vi "Init.vi"(8 "error in (no error)":errorcluster, 11 "Wifi in":refnum<class "Wifi.lvclass">) -> (0 "error out":errorcluster, 3 "Wifi out":refnum<class "Wifi.lvclass">)   [LabVIEW 2021, in "Wifi.lvclass"]
uses:
  Wifi.lvclass
  Wifi.lvclass/Wifi.ctl
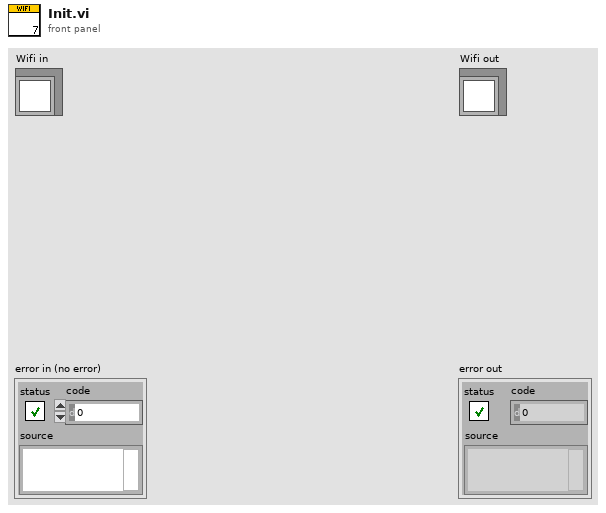
[diagram p1: front panel]
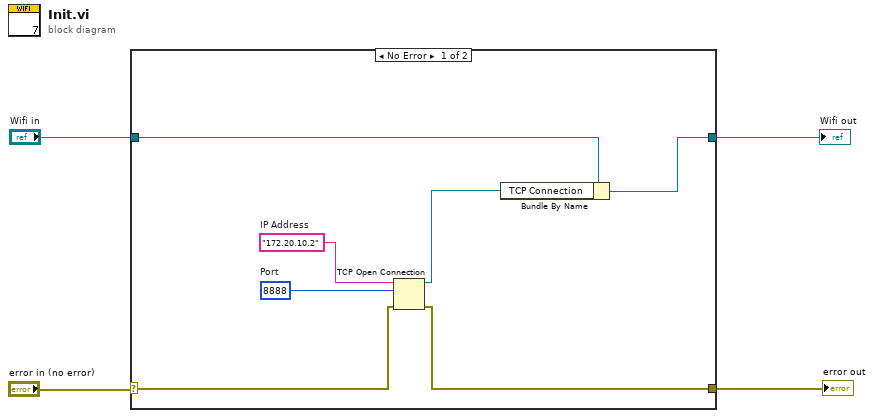
[diagram p0: block diagram]
diagram:
  n1 = case shown="No Error" "error in (no error)" {
    selector: "error in (no error)" -> [w9 w12]
    tunnel: [w8 w12] -> w3
    tunnel: [w5 w13] -> w2
    tunnel: "Wifi in" -> [w7 w13]
    frame No Error {
      w10 = u16 8888  # Port
      w11 = "172.20.10.2"  # IP Address
      n2 = TCP Open Connection(address=w11, remote port or service name=w10, error in (no error)=w9) -> (connection ID=w6:refnum<k5>, error out=w8:errorcluster)  [unwired: 2 in]
      n3 = Bundle By Name(cluster=w7, "TCP Connection"=w6) -> (w5:refnum<class "Wifi.lvclass">)
    }
    frame Error {
    }
  }
  "error out" <- w3
  "Wifi out" <- w2
